vi "High Level Cmd Interpreter.vi"(8 "Nominal Model param":T1={"za_true_0"=2.0, "za_work_0"=1.0, "zp_work_0"=-1.0, "zp_true_0"=-2.0, "IrisCenter_0"=[0.0, 5.0, 0.0]}, 11 "High Level cmd":T2={"za_true"=0.0, "za_work"=0.0, "zi"=0.0, "zp_work"=0.0, "zp_true"=0.0, "Iris XY Center"=[0.0, 5.0], "Iris XY Scaling"=[1.0, 1.0]}) -> (0 "Translation Array":dbl[](array[numeric]), 3 "Scaling Array":dbl[](array[numeric]), 4 "PC Displacement":dbl, 6 "AC Displacement":dbl)   [LabVIEW 2016]
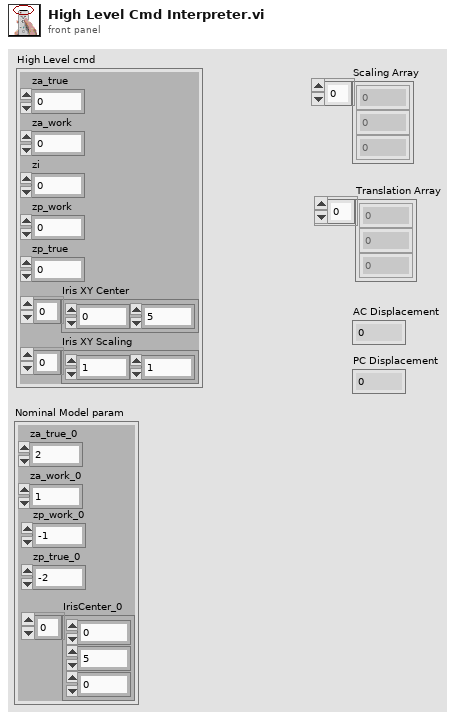
[diagram p1: front panel]
types:
  T1 = cluster{"za_true_0":dbl, "za_work_0":dbl, "zp_work_0":dbl, "zp_true_0":dbl, "IrisCenter_0":dbl[]}
  T2 = cluster{"za_true":dbl, "za_work":dbl, "zi":dbl, "zp_work":dbl, "zp_true":dbl, "Iris XY Center":dbl[], "Iris XY Scaling":dbl[]}
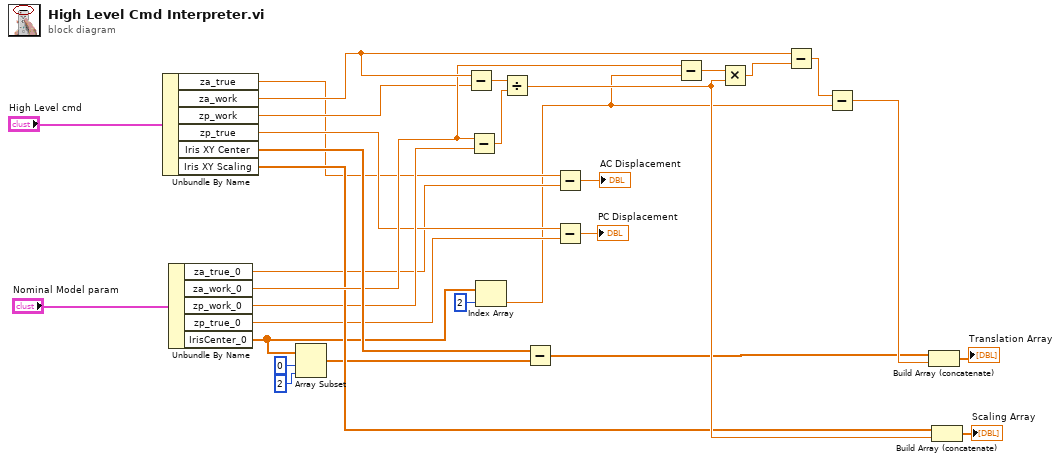
[diagram p0: block diagram]
diagram:
  n1 = Unbundle By Name("High Level cmd") -> ("za_true"=w5:dbl, "za_work"=w19:dbl, "zp_work"=w12:dbl, "zp_true"=w9:dbl, "Iris XY Center"=w18:dbl[], "Iris XY Scaling"=w16:dbl[])
  n2 = Unbundle By Name("Nominal Model param") -> ("za_true_0"=w4:dbl, "za_work_0"=w17:dbl, "zp_work_0"=w11:dbl, "zp_true_0"=w8:dbl, "IrisCenter_0"=w3:dbl[])
  n3 = Array Subset(array=w3, index=0, length=2) -> (w13:dbl[])
  n4 = Subtract(x=w19, y=w12) -> (x-y=w29:dbl)
  n5 = Subtract(x=w17, y=w11) -> (x-y=w7:dbl)
  n6 = Index Array(array=w3, index=2) -> (element=w1:dbl)
  n7 = Divide(x=w29, y=w7) -> (x/y=w24:dbl)
  n8 = Subtract(x=w18, y=w13) -> (x-y=w21:dbl[])
  n9 = Subtract(x=w5, y=w4) -> (x-y=→"AC Displacement":dbl)
  n10 = Subtract(x=w9, y=w8) -> (x-y=→"PC Displacement":dbl)
  n11 = Subtract(x=w17, y=w1) -> (x-y=w30:dbl)
  n12 = Multiply(x=w30, y=w24) -> (x*y=w28:dbl)
  n13 = Subtract(x=w19, y=w28) -> (x-y=w27:dbl)
  n14 = Subtract(x=w27, y=w1) -> (x-y=w22:dbl)
  n15 = Build Array (concatenate)(w21, w22) -> (→"Translation Array":dbl[])
  n16 = Build Array (concatenate)(w16, w24) -> (→"Scaling Array":dbl[])
